vi "Read Subscribe Set.vi"(8 "error in (no error)":errorcluster, 11 "Observer in":refnum<class "Observer.lvclass">) -> (0 "error out":errorcluster, 2 "Subscribe Set":T1, 3 "Observer out":refnum<class "Observer.lvclass">)   [LabVIEW 2019, in "Observer.lvclass"]
uses:
  Observer.lvclass
  Type Def/Subcribe Set.ctl
  Subscriber/Subscriber.lvclass
  Observer.lvclass/Observer.ctl
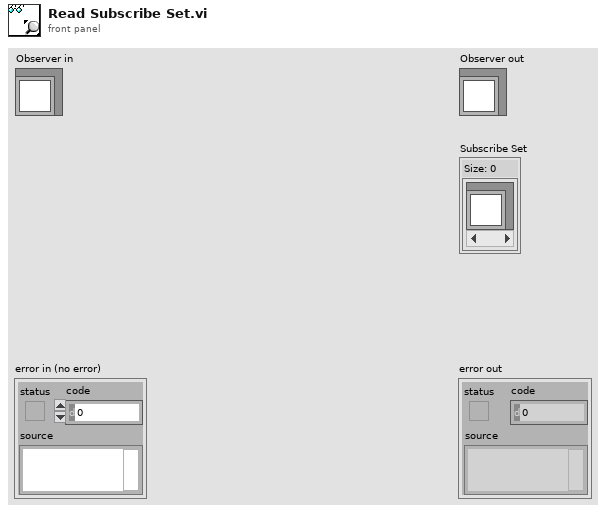
[diagram p1: front panel]
types:
  T1 = typedef "Subcribe Set.ctl" = set{refnum<class "Subscriber.lvclass">}
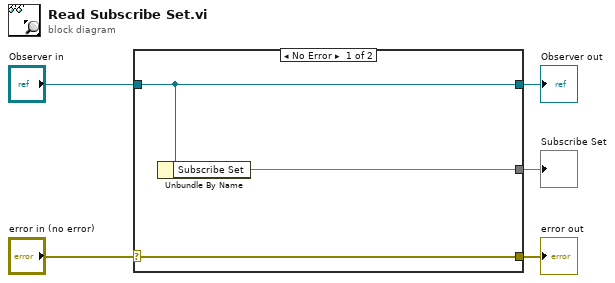
[diagram p0: block diagram]
diagram:
  n1 = case shown="No Error" "error in (no error)" {
    selector: "error in (no error)" -> [w8 w9]
    tunnel: [w8 w9] -> w4
    tunnel: [w7 w10] -> w2
    tunnel: "Observer in" -> [w7 w10]
    tunnel: [w6 _] -> w1
    frame No Error {
      n2 = Unbundle By Name(w7) -> ("Subscribe Set"=w6:T1)
    }
    frame Error {
    }
  }
  "error out" <- w4
  "Observer out" <- w2
  "Subscribe Set" <- w1
